vi "niRFUtil LCAPI Copy 1D Array (1 I32, 2 DBL).vi"(0 "Source0 1D Array (I32)":i32[](array[numeric]), 5 "Source1 1D Array (DBL)":dbl[](array[numeric]) format="%.2f", 7 "Source2 1D Array (DBL)":dbl[](array[numeric]) format="%.2f", 11 "error in (no error)":errorcluster, 12 "Data Copy Descriptor":u64) -> (4 "Source0 Out":i32[](array[numeric]), 6 "Source1 Out":dbl[](array[numeric]) format="%.2f", 8 "Source2 Out":dbl[](array[numeric]) format="%.2f", 15 "error out":errorcluster)   [LabVIEW 2015, in "niRFUtil.lvlib"]
uses:
  niRFUtil.lvlib
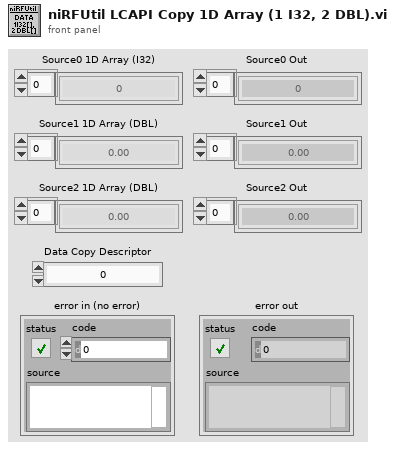
[diagram p1: front panel]
types:
  T1 = cluster{"status":bool, "return type":i32, "errorString":string}
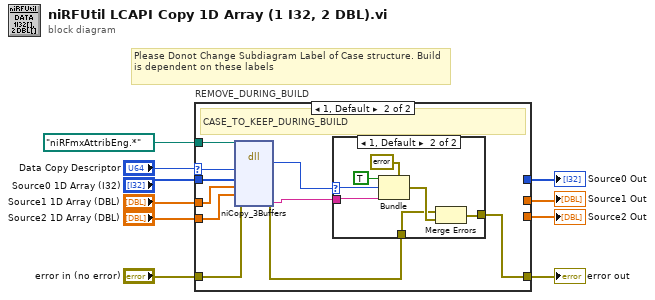
[diagram p0: block diagram]
diagram:
  # "Please Donot Change Subdiagram Label of Case structure. Build is dependent on these labels"
  n1 = case "REMOVE_DURING_BUILD" shown="1, Default" "Data Copy Descriptor" {
    selector: "Data Copy Descriptor" -> [_ w16]
    tunnel: "error in (no error)" -> [w11 w23]
    tunnel: "Source1 1D Array (DBL)" -> [w13 w22]
    tunnel: "Source2 1D Array (DBL)" -> [w12 w21]
    tunnel: "Source0 1D Array (I32)" -> [w14 w20]
    tunnel: [w14 _] -> w4
    tunnel: [w13 _] -> w5
    tunnel: [w12 _] -> w3
    tunnel: [w11 w24] -> w2
    tunnel: path "niRFmxAttribEng.*" ("path in") -> [_ w15]
    frame 0 {
      # "Development"
    }
    frame 1, Default {
      # "CASE_TO_KEEP_DURING_BUILD"
      n2 = dll-call lib="niRFmxAttribEng.*" fn="niCopy_3Buffers"(path in=w15, error in=w23, "dataCopyDescriptor"=w16, "source0"=w20, "source1"=w22, "source2"=w21) -> (error out=w17:errorcluster, "return type"=w19:i32, "errorString"=w18:string)  [unwired: 6 in, 1 out]
      n3 = case shown="1, Default" w19 {
        selector: w19 -> [_ w31]
        tunnel: w18 -> [_ w30]
        tunnel: w17 -> [w25 w26]
        tunnel: [w25 w29] -> w24
        frame 0 {
        }
        frame 1, Default {
          n4 = Bundle(cluster=T1 {"status"=FALSE, "return type"=0, "errorString"=""}, "status"=TRUE, "return type"=w31, "errorString"=w30) -> (w28:T1)
          n5 = Merge Errors(w26, w28) -> (w29:errorcluster)
        }
      }
    }
  }
  "error out" <- w2
  "Source0 Out" <- w4
  "Source1 Out" <- w5
  "Source2 Out" <- w3
